vi "LabVIEW_program.vi"() -> ()   [LabVIEW 2022 SP3]
uses:
  <vilib>/DAQmx/read.llb/DAQmx Read (Analog 1D DBL NChan 1Samp).vi
  <vilib>/DAQmx/create/channels.llb/DAQmx Create Channel (AI-Voltage-Basic).vi
  <vilib>/DAQmx/miscellaneous.llb/DAQmx Fill In Error Info.vi
panel:
  out "weight voltage":dbl
  out "Waveform Chart":dbl(graph)
  in  "VISA resource name 2":refnum<visa-resource-name>
  in  "VISA resource name":refnum<visa-resource-name>
  in  "physical channels":tag
  in  "stop":bool
  out "humidity":dbl
  in  "Voltage threshold":dbl
  out "?":bool
  out "Counter":dbl
  out "voltage":dbl
  out "weight":dbl
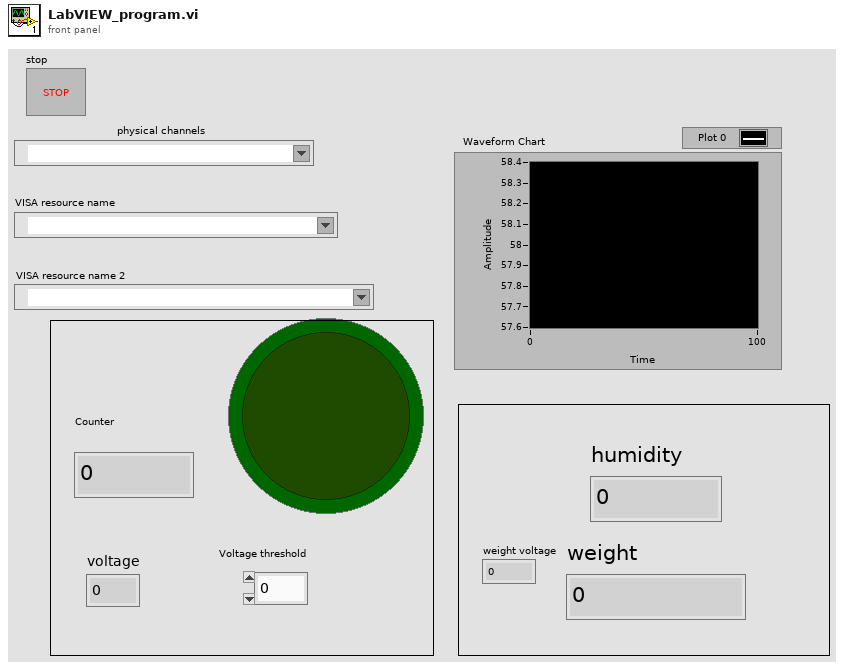
[diagram p1: front panel]
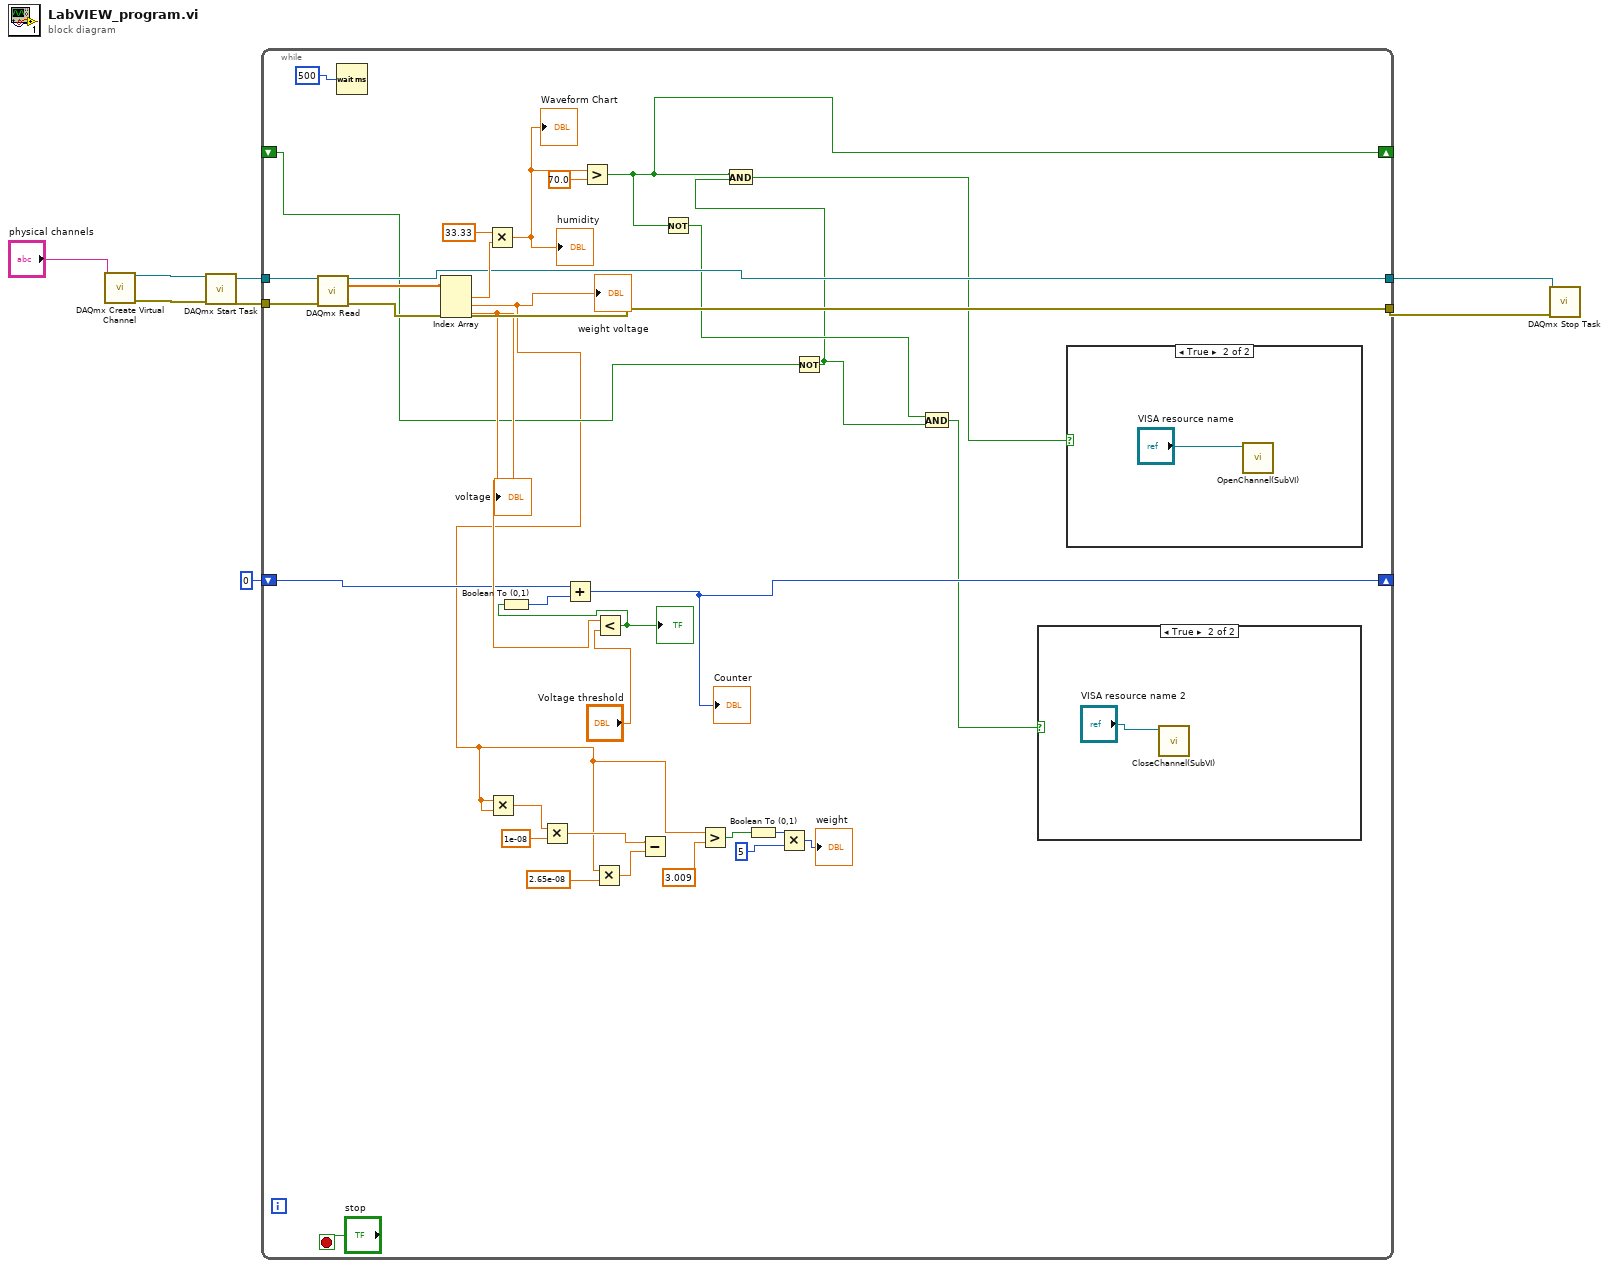
[diagram p0: block diagram]
diagram:
  n1 = call-poly <vilib>:"DAQmx Create Virtual Channel.vi"("physical channels"="physical channels") -> ("task out"=w8:refnum<k21>, "error out"=w7:errorcluster)  [unwired: 13 in]
  n2 = call <vilib>:"DAQmx Start Task.vi"("task/channels in"=w8, "error in"=w7) -> ("task out"=w6:refnum<k21>, "error out"=w5:errorcluster)  [unwired: 12 in]
  n3 = while {
    tunnel: w6 -> [w42]
    tunnel: w5 -> [w41]
    tunnel: [w33] -> w4
    tunnel: [w34] -> w2
    shift-right: [w28] -> _
    shift-left: i16 0 -> [w27]
    shift-right: [w22] -> _
    shift-left: _ -> [w20]
    stop <- "stop" stop-if-true
    n4 = call-poly <vilib>:"DAQmx Read.vi"("task/channels in"=w42, "error in"=w41) -> ("task out"=w33:refnum<k21>, "data"=w38:dbl[], "error out"=w34:errorcluster)  [unwired: 11 in]
    n5 = Wait (ms)(milliseconds to wait=u32 500) -> ()  [unwired: 1 out]
    n6 = Index Array(array=w38) -> (element #1=w37:dbl, element #2=w14:dbl, element #3=w29:dbl)  [unwired: 3 in]
    "voltage" <- w29
    "weight voltage" <- w14
    n7 = Multiply(x=33.33, y=w37) -> (x*y=w15:dbl)
    "humidity" <- w15
    "Waveform Chart" <- w15
    n8 = Multiply(x=w14, y=w14) -> (x*y=w16:dbl)
    n9 = Multiply(x=w16, y=1e-08) -> (x*y=w24:dbl)
    n10 = Greater?(x=w15, y=70.0) -> (0:w22:bool)
    n11 = Multiply(x=w14, y=2.65e-08) -> (x*y=w23:dbl)
    n12 = Less?(x=w29, y="Voltage threshold") -> (x < y?=w30:bool)
    "?" <- w30
    n13 = Boolean To (0,1)(Boolean=w30) -> (0, 1=w31:i16)
    n14 = Add(x=w27, y=w31) -> (x+y=w28:i16)
    "Counter" <- w28
    n15 = Subtract(x=w24, y=w23) -> ()  [unwired: 1 out]
    n16 = Not(x=w22) -> (.not. x?=w21:bool)
    n17 = Greater?(x=w14, y=3.009) -> (0:w12:bool)
    n18 = Boolean To (0,1)(Boolean=w12) -> (0, 1=w11:i16)
    n19 = Multiply(x=w11, y=i16 5) -> (x*y=→"weight":i16)
    n20 = Not(x=w20) -> (.not. x?=w17:bool)
    n21 = And(x=w22, y=w17) -> (x .and. y?=w19:bool)
    n22 = And(x=w21, y=w17) -> (x .and. y?=w18:bool)
    n23 = case shown="True" w18 {
      frame False {
      }
      frame True {
        n24 = call "CloseChannel(SubVI).vi"("VISA Refnum in"="VISA resource name 2") -> ()  [unwired: 11 in]
      }
    }
    n25 = case shown="True" w19 {
      frame False {
      }
      frame True {
        n26 = call "OpenChannel(SubVI).vi"("VISA Refnum in"="VISA resource name") -> ()  [unwired: 11 in]
      }
    }
  }
  n27 = call <vilib>:"DAQmx Stop Task.vi"("task/channels in"=w4, "error in"=w2) -> ()  [unwired: 12 in, 2 out]
